vi "CheckAstromechState.vi"(8 "Error In":errorcluster, 10 "With sound?":bool, 11 "Astromech droid In":refnum<class "Astromech droid.lvclass">) -> (0 "Error Out":errorcluster, 3 "Astromech droid Out":refnum<class "Astromech droid.lvclass">)   [LabVIEW 2021, in "Astromech droid.lvclass"]
doc: "Show visual and optional sound information about astromech active state."
uses:
  Astromech droid.lvclass
  Astromech droid.lvclass/Astromech droid.ctl
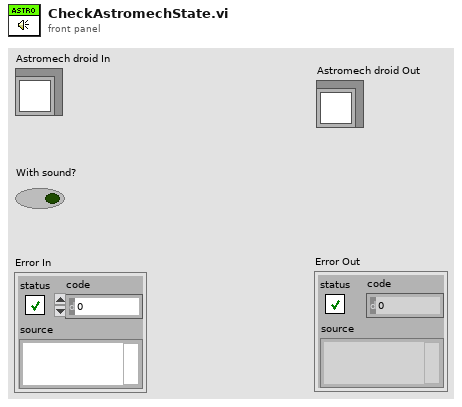
[diagram p1: front panel]
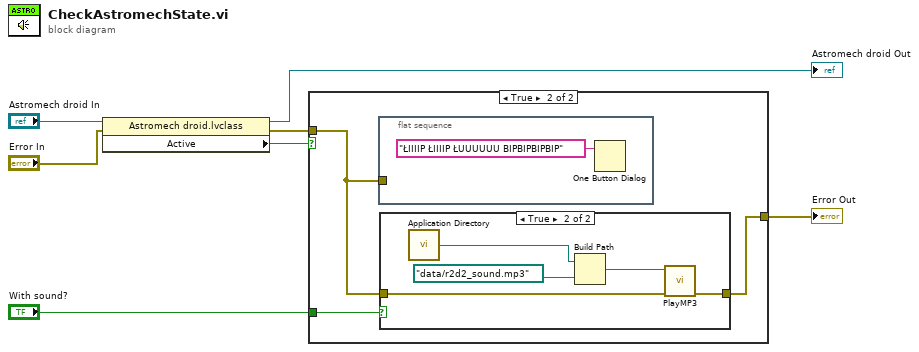
[diagram p0: block diagram]
diagram:
  n1 = property class="Astromech droid.lvclass"(reference="Astromech droid In", error in="Error In") -> (reference out=→"Astromech droid Out":refnum<class "Astromech droid.lvclass">, error out=w1:errorcluster, "Active"=w4:bool)
  n2 = case shown="True" w4 {
    tunnel: [w8 w11] -> w7
    tunnel: "With sound?" -> [_ w10]
    tunnel: w1 -> [w8 w9]
    frame False {
    }
    frame True {
      n3 = flat-sequence {
        tunnel: w9 -> [_]
        frame #0 {
          n4 = One Button Dialog(message="ŁIIIIP ŁIIIIP ŁUUUUUU BIPBIPBIPBIP") -> ()  [unwired: 1 in, 1 out]
        }
      }
      n5 = case shown="True" w10 {
        tunnel: w9 -> [w13 w15]
        tunnel: [w13 w14] -> w11
        frame False {
        }
        frame True {
          n6 = call <vilib>:"Application Directory.vi"() -> ("Application Directory"=w16:path)
          n7 = Build Path(base path=w16, name or relative path=path "data/r2d2_sound.mp3") -> (appended path=w18:path)
          n8 = call "PlayMP3.vi"("Error In"=w15, "Path"=w18) -> ("Error out"=w14:errorcluster)  [unwired: 9 in]
        }
      }
    }
  }
  "Error Out" <- w7
